vi "Test Jobber.vi"   [LabVIEW 2014]
uses:
  Core/LabVIEW CI Service/Actors/Jobber/Jobber/Jobber.lvclass
  Dummy Job/Dummy Job.lvclass
  Core/LabVIEW CI Service/Actors/Jobber/Jobber/Jobber.lvclass/Jobber.ctl
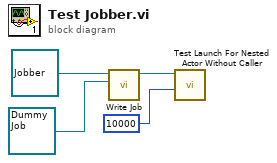
[diagram p0: block diagram]
diagram:
  n1 = call "Write Job.vi"("Job.lvclass"=refnum<class "Dummy Job.lvclass"> refnum ("Dummy Job.lvclass"), "Jobber in"=refnum<class "Jobber.lvclass"> refnum ("Jobber.lvlib:Jobber.lvclass")) -> ("Jobber out"=w2:refnum<class "Jobber.lvclass">)  [unwired: 9 in]
  n2 = call "Test Launch For Nested Actor Without Caller.vi"("timeout in ms (-1)"=10000, "Actor Before Launch"=w2) -> ()  [unwired: 8 in, 2 out]
